vi "open_loop.vi"() -> ()   [LabVIEW 2015]
panel:
  out "Waveform Chart":dbl(graph)
  in  "Alerta N. Bajo":dbl=10.0 min=10.0 max=50.0
  in  "Alerta N. Alto":dbl=50.0 min=50.0 max=90.0
  out "Alert. N. Bajo":bool
  out "Alert. N. Alto":bool
  out "% 2":dbl
  out "%":dbl
  in  "V. Inicial":dbl
  out "V. Entrada":bool
  out "V. Salida":bool
  in  "Nivel de Apert. Salida %":dbl(knob) scale=0.0..1.0
  in  "Nivel de Apert. Entrada %":dbl(knob) scale=0.0..1.0
  in  "Controles":T1
  in  "Stop":bool
  out "Nivel de Tanque":dbl(knob) scale=0.0..100.0
  out "Nivel de Tanque %":dbl
  out "Tanque":dbl(slide) scale=0.0..100.0
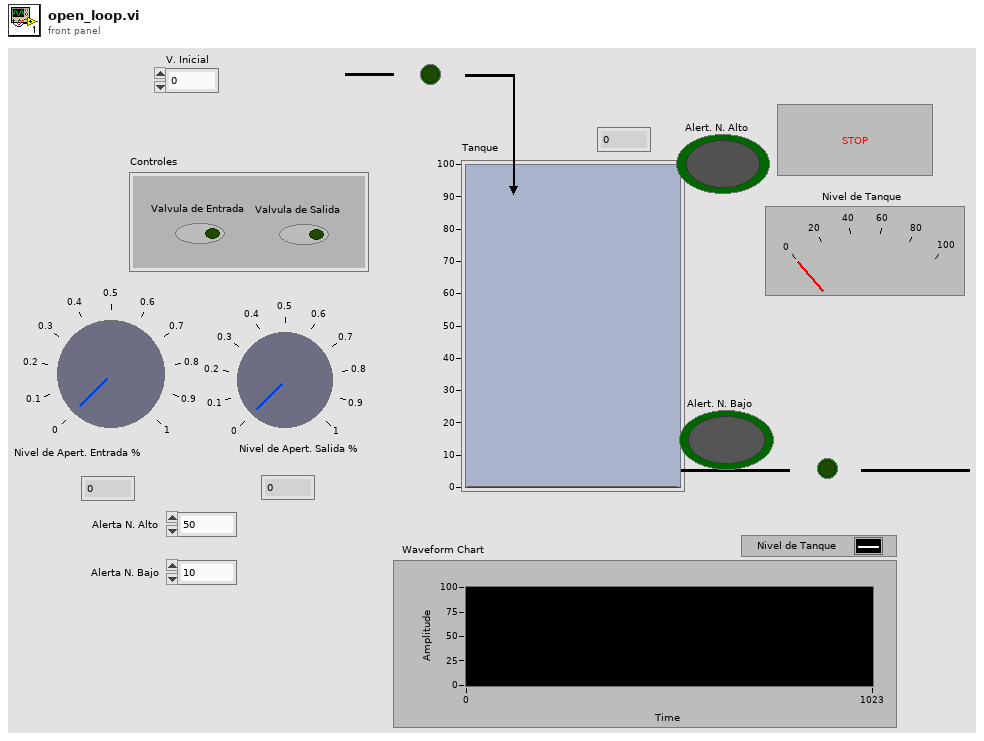
[diagram p1: front panel]
types:
  T1 = cluster{"Valvula de Entrada":bool, "Valvula de Salida":bool}
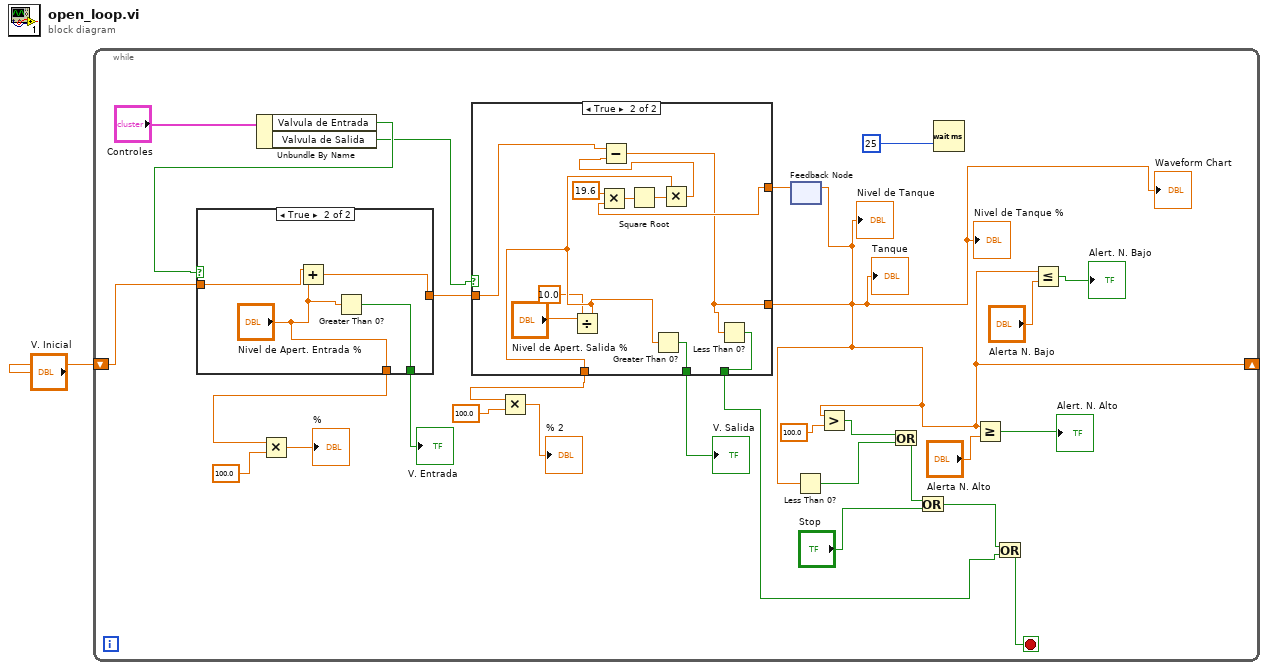
[diagram p0: block diagram]
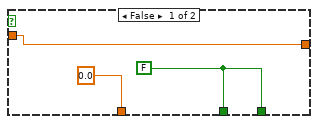
[diagram p2: hidden frame]
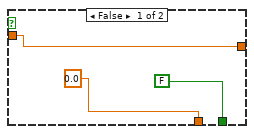
[diagram p3: hidden frame]
diagram:
  n1 = while {
    shift-right: [w2] -> _
    shift-left: "V. Inicial" -> [w26]
    stop <- w3 stop-if-true
    n2 = Unbundle By Name("Controles") -> ("Valvula de Entrada"=w27:bool, "Valvula de Salida"=w24:bool)
    n3 = case shown="True" w27 {
      tunnel: w26 -> [w47 w50]
      tunnel: [w47 w51] -> w25
      tunnel: [FALSE w49] -> w18
      tunnel: [0.0 "Nivel de Apert. Entrada %"] -> w16
      frame False {
      }
      frame True {
        n4 = Add(x=w50, y="Nivel de Apert. Entrada %") -> (x+y=w51:dbl)
        n5 = Greater Than 0?(x="Nivel de Apert. Entrada %") -> (x > 0?=w49:bool)
      }
    }
    "V. Entrada" <- w18
    n6 = Multiply(x=w16, y=100.0) -> (x*y=→"%":dbl)
    n7 = feedback #1() -> (w6:dbl)  [unwired: 1 in]
    n8 = case shown="True" w24 {
      tunnel: w25 -> [w32 w44]
      tunnel: [w32 w37] -> w2
      tunnel: [w30 w43] -> w17
      tunnel: [0.0 w35] -> w12
      tunnel: w6 -> [_ w38]
      tunnel: [w30 w36] -> w4
      frame False {
        w30 = FALSE
      }
      frame True {
        n9 = Divide(x="Nivel de Apert. Salida %", y=10.0) -> (x/y=w35:dbl)
        n10 = Multiply(x=19.6, y=w38) -> (x*y=w41:dbl)
        n11 = Square Root(x=w41) -> (sqrt(x)=w42:dbl)
        n12 = Greater Than 0?(x=w35) -> (x > 0?=w43:bool)
        n13 = Multiply(x=w35, y=w42) -> (x*y=w39:dbl)
        n14 = Subtract(x=w44, y=w39) -> (x-y=w37:dbl)
        n15 = Less Than 0?(x=w37) -> (x < 0?=w36:bool)
      }
    }
    "Tanque" <- w2
    "Nivel de Tanque %" <- w2
    "Nivel de Tanque" <- w2
    "V. Salida" <- w17
    "Waveform Chart" <- w2
    n16 = Multiply(x=w12, y=100.0) -> (x*y=→"% 2":dbl)
    n17 = feedback-in #1(w2) -> ()
    n18 = Less Than 0?(x=w2) -> (x < 0?=w20:bool)
    n19 = Greater?(x=w2, y=100.0) -> (0:w21:bool)
    n20 = Or(x=w21, y=w20) -> (x .or. y?=w19:bool)
    n21 = Or(x=w19, y="Stop") -> (x .or. y?=w5:bool)
    n22 = Wait (ms)(milliseconds to wait=25) -> ()  [unwired: 1 out]
    n23 = Greater Or Equal?(x=w2, y="Alerta N. Alto") -> (x >= y?=→"Alert. N. Alto":bool)
    n24 = Or(x=w5, y=w4) -> (x .or. y?=w3:bool)
    n25 = Less Or Equal?(x=w2, y="Alerta N. Bajo") -> (x <= y?=→"Alert. N. Bajo":bool)
  }
